vi "Read Waveform Core.vi"(0 "IVI_Scope in":refnum<class "IVI_Scope.lvclass">, 1 "channel name (\"CHANNEL1\")":string="CHANNEL1", 2 "maximum time (5000ms)":i32=5000, 3 "waveform size (0)":i32=1000 caption="waveform size (1000)", 5 "error in (no error)":errorcluster) -> (14 "IVI_Scope out":refnum<class "IVI_Scope.lvclass">, 15 "waveform array":dbl[unit][](array[numeric]) format="%.3f", 16 "actual points":i32, 17 "initial x":dbl[unit] caption="initial x (seconds)" format="%^.2e", 18 "x increment":dbl[unit] caption="x increment (seconds)" format="%^.2e", 19 "error out":errorcluster)   [LabVIEW 2016, in "IVI_Scope.lvlib" / "IVI_Scope.lvclass"]
doc: "This VI initiates an acquisition on all channels that you enable with the IviScope Configure Channel VI. If the channel you specify in the Channel Name parameter is not enabled for the acquisition, this VI returns the IVISCOPE_ERROR_CHANNEL_NOT_ENABLED (0xBFFA2001) error. It then waits for the acquisition to complete and returns the waveform for the channel you specify. If the oscilloscope did not complete the acquisition within the time period you specify with the Maximum Time parameter, the VI returns the IVISCOPE_ERROR_MAX_TIME_EXCEEDED (0xBFFA2003) error.\n\nYou call the IviScope Fetch Waveform VI to obtain the waveforms for each of the remaining enabled channels without initiating another acquisition.\n\nNotes:\n \n(1) Use this VI to read waveforms when you set the acquisition mode to IVISCOPE_VAL_NORMAL, IVISCOPE_VAL_HI_RES, or IVISCOPE_VAL_AVERAGE. If the acquisition type is not one of the listed types, the VI returns the IVISCOPE_ERROR_INVALID_ACQ_TYPE (0xBFFA2004) error.\n\n(2) After this VI executes, each element in the Waveform Array parameter is either a voltage or a value indicating that the oscilloscope could not sample a voltage.\n\n(3) You configure the interpolation method the oscilloscope uses with the IviScope Is Invalid Waveform Element VI. If you disable interpolation, the oscilloscope does not interpolate points in the waveform. If the oscilloscope cannot sample a value for a point in the waveform, the driver sets the corresponding element in the Waveform Array to an IEEE defined NaN (Not a Number) value and the VI returns IVISCOPE_WARN_INVALID_WFM_ELEMENT (0x3FFA2001).\n\n(4) You can test a waveform value for an invalid value condition by calling the IviScope Is Invalid Waveform Element VI.\n\n(5) This VI performs interchangeability checking when the IviScope>>Inherent IVI Settings>>User Options>>Interchange Check property is set to TRUE. If the IviScope>>Inherent IVI Settings>>User Options>>Spy property is set to TRUE, you use the NI I/O Trace utility to view interchangeability warnings. You use the IviScope Get Next Interchange Warning VI to retrieve interchangeability warnings when the IviScope>>Inherent IVI Settings>>User Options>>Spy property is set to FALSE. For more information about interchangeability checking, refer to the help text for the IviScope>>Inherent IVI Settings>>User Options>>Interchange Check property.\n\n(6) The class driver returns a simulated waveform when this VI is called and the IviScope>>Inherent IVI Settings>>User Options>>Simulate property is set to TRUE and the IviScope>>Inherent IVI Settings>>User Options>>Use Specific Simulation property is set to FALSE. For information on how to configure a simulated waveform, refer to the online help manual."
uses:
  IVI_Scope.lvclass
  IVI_Scope.lvclass/IVI_Scope.ctl
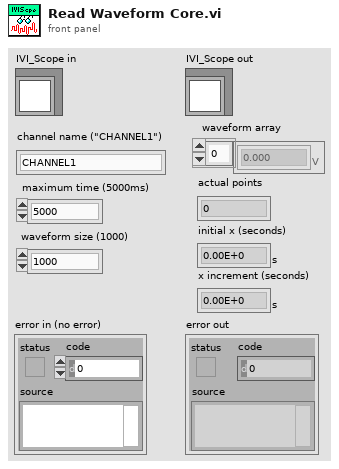
[diagram p1: front panel]
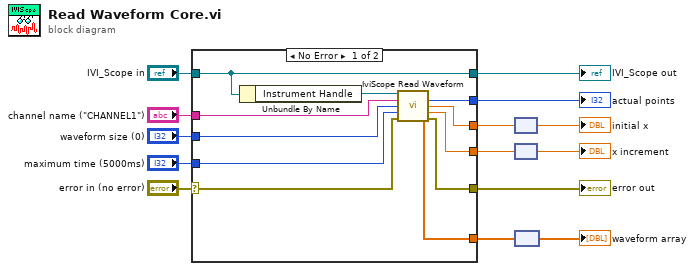
[diagram p0: block diagram]
diagram:
  n1 = case shown="No Error" "error in (no error)" {
    selector: "error in (no error)" -> [w20 w27]
    tunnel: [w19 w27] -> w13
    tunnel: [w25 w26] -> w11
    tunnel: "IVI_Scope in" -> [w25 w26]
    tunnel: "channel name (\"CHANNEL1\")" -> [w23 _]
    tunnel: "waveform size (0)" -> [w22 _]
    tunnel: "maximum time (5000ms)" -> [w21 _]
    tunnel: [w18 _] -> w2
    tunnel: [w17 _] -> w7
    tunnel: [w16 _] -> w6
    tunnel: [w15 _] -> w5
    frame No Error {
      n2 = Unbundle By Name(w25) -> ("Instrument Handle"=w24:refnum<k15>)
      n3 = call <vilib>:"IviScope Read Waveform.vi"("instrument handle"=w24, "channel name (\"CHANNEL1\")"=w23, "waveform size (0)"=w22, "maximum time (5000ms)"=w21, "error in (no error)"=w20) -> ("actual points"=w17:i32, "initial x"=w16:dbl, "x increment"=w15:dbl, "waveform array"=w18:dbl[], "error out"=w19:errorcluster)  [unwired: 5 in, 1 out]
    }
    frame Error {
    }
  }
  "error out" <- w13
  "IVI_Scope out" <- w11
  "actual points" <- w7
  n4 = node(w6) -> (→"initial x":dbl[unit])
  n5 = node(w5) -> (→"x increment":dbl[unit])
  n6 = node(w2) -> (→"waveform array":dbl[unit][])
